vi "RT Main5.vi"() -> ()   [LabVIEW 2019]
uses:
  <vilib>/FPGAPlugInAG/ELVIS III/niLvFpga_Open_ELVIS III.vi
  <vilib>/rvi/interface/common/dynamic/niFpgaDynamicAddResources.vi
  <vilib>/myRIO/Common/Instrument Driver Framework/Utilities/vis/FPGA Ref Manager.vi
  <vilib>/Utility/error.llb/Error Cluster From Error Code.vi
  <vilib>/myRIO/Common/Instrument Driver Framework/Utilities/vis/Ref Counter.vi
  <vilib>/rvi/errors/niLvFpgaAdjustHostInterfaceError.vi
  <vilib>/FPGAPlugInAG/Dynamic/niLvFpga_Close_Dynamic.vi
  <vilib>/rvi/interface/nirviOpenFPGA/nirviOpenFPGA.xnode
  FPGA Bitfiles/measurementpwmfr_FPGATarget_PWM5_dVHC8fwqfPA.lvbitx
  PWM5.vi
  <vilib>/rvi/interface/nirviReadWriteControl/nirviReadWriteControl.xnode
  <vilib>/rvi/interface/nirviCloseFPGA/nirviCloseFPGA.xnode
  <vilib>/myRIO/Instrument Drivers/Utilities/Utilities.lvlib
  NiFpgaLv.dll
  <vilib>/rvi/interface/Simulation/niFpgaSimulationCallBeginRW.vi
panel:
  out "Error":dbl
  out "error out":errorcluster
  in  "Stop":bool
  out "波形图表":dbl(graph)
  out "数值":dbl format="%#_16g"
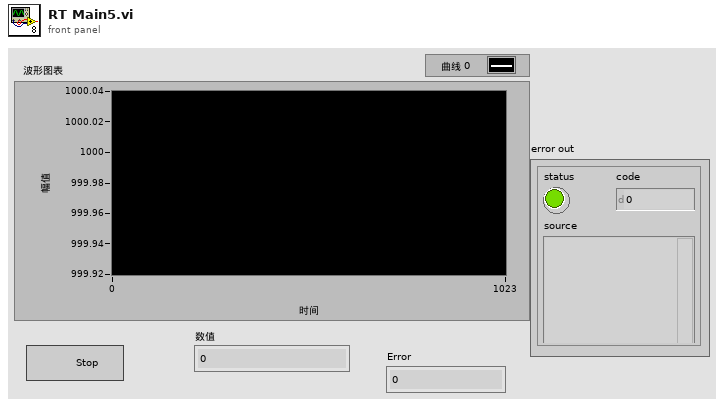
[diagram p1: front panel]
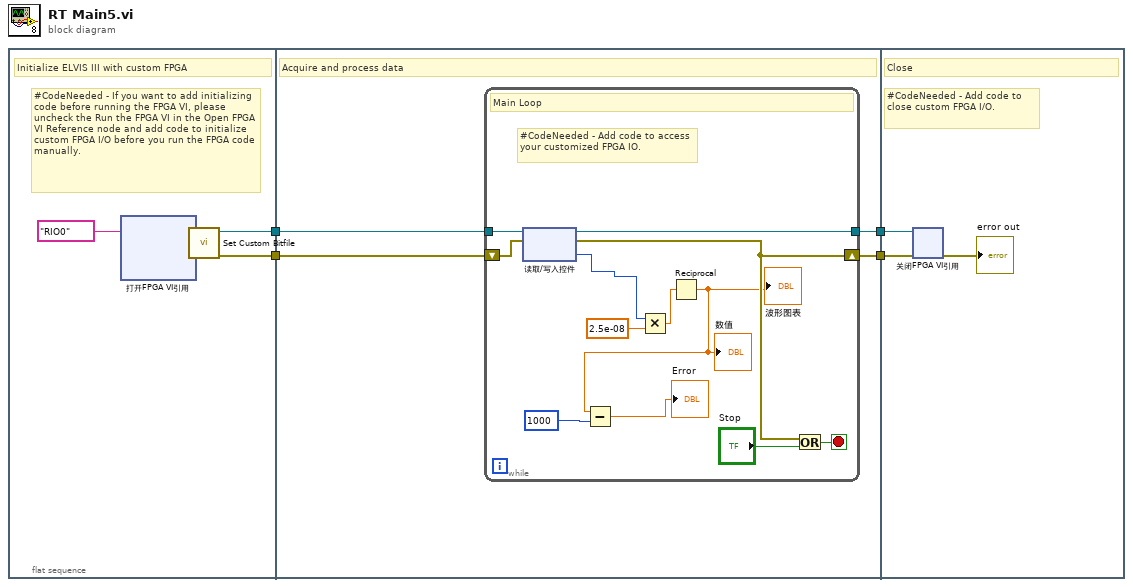
[diagram p0: block diagram]
diagram:
  n1 = flat-sequence {
    tunnel: [w6] -> w4
    tunnel: [w7] -> w3
    tunnel: w4 -> [w13]
    tunnel: w3 -> [w12]
    tunnel: [w11] -> w2
    tunnel: [w10] -> w1
    tunnel: w2 -> [w28]
    tunnel: w1 -> [w27]
    frame #0 {
      # "#CodeNeeded - If you want to add initializing code before running the FPGA VI, please uncheck the Run the FPGA VI in the Open FPGA VI Reference node and add code to initialize custom FPGA I/O before you run the FPGA code manually."
      # "Initialize ELVIS III with custom FPGA"
      n2 = xnode "打开FPGA VI引用"("资源名称"=tag "RIO0" ("resource name")) -> ("FPGA VI引用输出"=w8:refnum<k20>, "错误输出"=w9:errorcluster)  [unwired: 1 in]
      n3 = call <vilib>:"Set Custom Bitfile.vi"("error in (no error)"=w9, "Custom FPGA Reference In"=w8) -> ("error out"=w6:errorcluster, "Custom FPGA Reference Out"=w7:refnum<k20>)  [unwired: 8 in]
    }
    frame #1 {
      # "Acquire and process data"
      n4 = while {
        tunnel: w12 -> [w23]
        tunnel: [w22] -> w11
        shift-right: [w20] -> w10
        shift-left: w13 -> [w21]
        stop <- w24 stop-if-true
        # "#CodeNeeded - Add code to access your customized FPGA IO."
        # "Main Loop"
        n5 = xnode "读取/写入控件"("FPGA VI引用输入"=w23, "错误输入"=w21) -> ("FPGA VI引用输出"=w22:refnum<k20>, "错误输出"=w20:errorcluster, "x-1"=w17:u32)
        n6 = Multiply(x=w17, y=2.5e-08) -> (x*y=w19:dbl)
        n7 = Reciprocal(x=w19) -> (1/x=w16:dbl)
        "波形图表" <- w16
        "数值" <- w16
        n8 = Subtract(x=w16, y=u32 1000) -> (x-y=→"Error":dbl)
        n9 = Or(x=w20, y="Stop") -> (x .or. y?=w24:bool)
      }
    }
    frame #2 {
      # "#CodeNeeded - Add code to close custom FPGA I/O."
      # "Close"
      n10 = xnode "关闭FPGA VI引用"("FPGA VI引用输入"=w28, "错误输入"=w27) -> ("错误输出"=→"error out":errorcluster)
    }
  }
